vi "Parse.vi"(8 "error in (no error)":errorcluster, 10 "Properties String":string, 11 "CSSProperties in":refnum<class "CSSProperties.lvclass">) -> (0 "error out":errorcluster, 2 "KVPs":cluster{"Properties":string, "Values":string}[](array[cluster]), 3 "CSSProperties out":refnum<class "CSSProperties.lvclass">)   [LabVIEW 2019, in "CSSProperties.lvclass"]
uses:
  CSSProperties.lvclass
  <vilib>/Utility/error.llb/whitespace.ctl
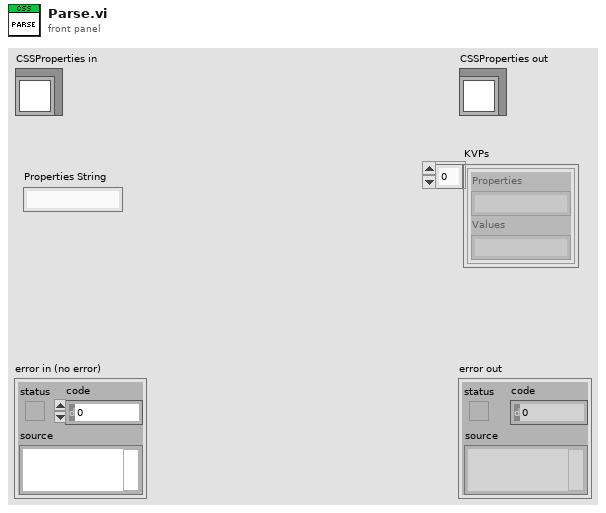
[diagram p1: front panel]
types:
  T1 = typedef "whitespace.ctl" = u16
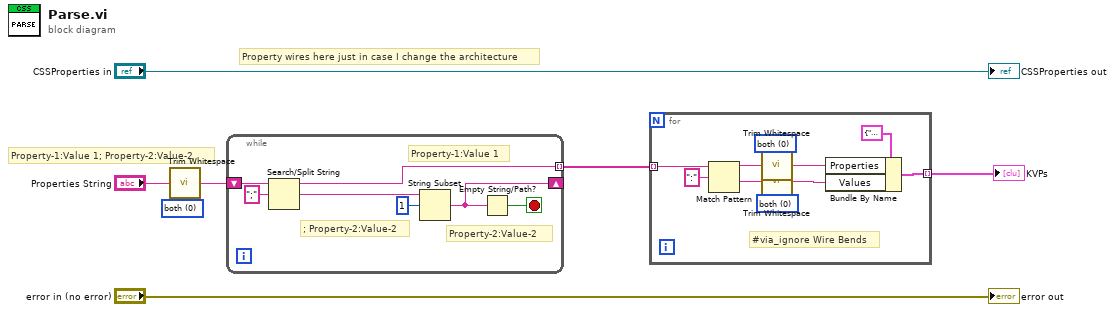
[diagram p0: block diagram]
diagram:
  w4 = T1 0 items=["both", "start of string", "end of string"] ("location (both)")
  # "Property wires here just in case I change the architecture"
  # "Property-1:Value 1; Property-2:Value-2"
  n1 = call <vilib>:"Trim Whitespace.vi"("string"="Properties String", "location (both)"=w4) -> ("trimmed string"=w3:string)
  n2 = while {
    shift-right: [w9] -> _
    shift-left: w3 -> [w14]
    tunnel: [w8] -> w2 mode=indexing
    stop <- w10 stop-if-true
    # "Property-2:Value-2"
    # "; Property-2:Value-2"
    # "Property-1:Value 1"
    n3 = Search/Split String(string=w14, search string/char (-)=";") -> (substring before match=w8:string, match + rest of string=w12:string)  [unwired: 1 in, 1 out]
    n4 = String Subset(string=w12, offset (0)=1) -> (substring=w9:string)  [unwired: 1 in]
    n5 = Empty String/Path?(string/path=w9) -> (empty?=w10:bool)
  }
  n6 = for {
    tunnel: w2 -> [w24] mode=indexing
    tunnel: [w15] -> w1 mode=indexing
    w19 = T1 0 items=["both", "start of string", "end of string"] ("location (both)")
    w22 = T1 0 items=["both", "start of string", "end of string"] ("location (both)")
    # "#via_ignore Wire Bends"
    n7 = Match Pattern(string=w24, regular expression=":") -> (before substring=w21:string, after substring=w20:string)  [unwired: 1 in, 2 out]
    n8 = call <vilib>:"Trim Whitespace.vi"("string"=w21, "location (both)"=w22) -> ("trimmed string"=w17:string)
    n9 = call <vilib>:"Trim Whitespace.vi"("string"=w20, "location (both)"=w19) -> ("trimmed string"=w16:string)
    n10 = Bundle By Name(cluster=cluster{"Properties":string, "Values":string} {"Properties"="", "Values"=""} ("Pair"), "Properties"=w17, "Values"=w16) -> (w15:cluster{"Properties":string, "Values":string})
  }
  "KVPs" <- w1
  "error out" <- "error in (no error)"
  "CSSProperties out" <- "CSSProperties in"
